vi "HH_Init.vi"(0 "MAXDEV":i32=8, 11 "error in (no error)":errorcluster) -> (4 "Library Version":string="2.1", 6 "Device List":T1(array[cluster]), 15 "error out":errorcluster)   [LabVIEW 2013]
doc: "Prepare PicoHarp 300 for T3R-Measurement"
uses:
  MT Scan/SubVIs/hhlib.dll
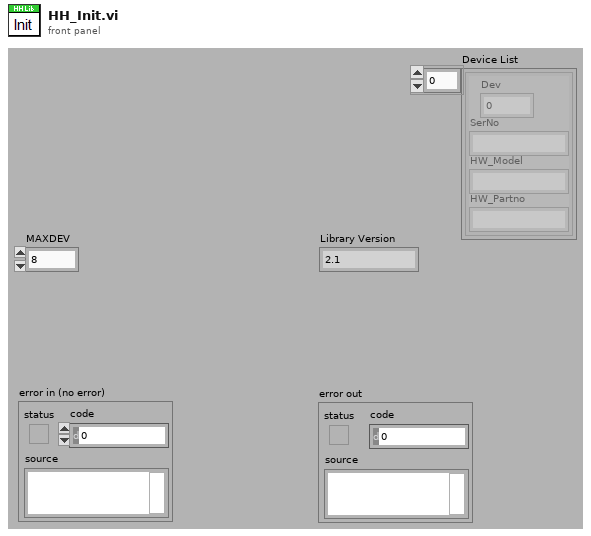
[diagram p1: front panel]
types:
  T1 = cluster{"Dev":i32, "SerNo":string, "HW_Model":string, "HW_Partno":string}[]
  T2 = cluster{"Dev":i32, "SerNo":string, "HW_Model":string, "HW_Partno":string}
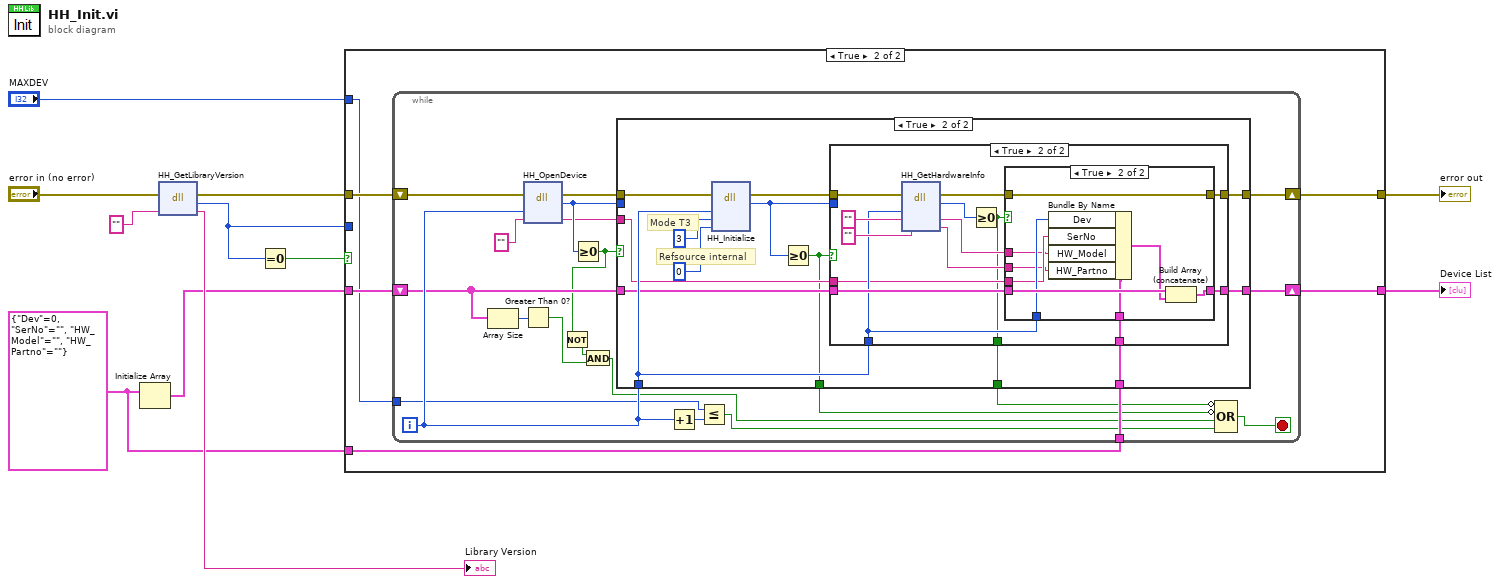
[diagram p0: block diagram]
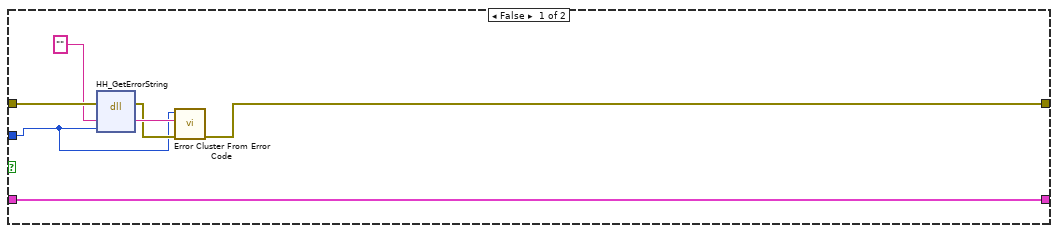
[diagram p2: hidden frame]
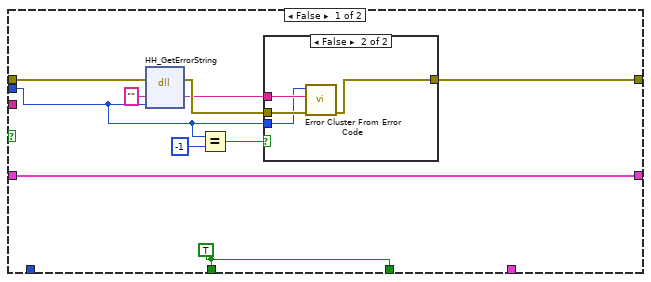
[diagram p3: hidden frame]
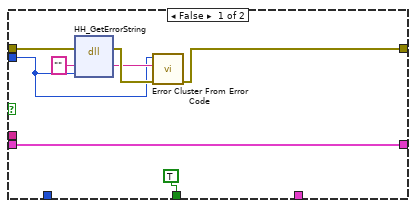
[diagram p5: hidden frame]
diagram:
  w2 = T2 {"Dev"=0, "SerNo"="", "HW_Model"="", "HW_Partno"=""}
  n1 = Initialize Array(w2) -> (w3:T1)  [unwired: 1 in]
  n2 = dll-call lib="C:/Users/dhaehnel/Documents/Workspace/Labview_Workspace/newCore/MT Scan/SubVIs/hhlib.dll" fn="HH_GetLibraryVersion"(error in="error in (no error)", "vers"="") -> (error out=w8:errorcluster, "return type"=w4:i32, "vers"=→"Library Version":string)  [unwired: 2 in, 1 out]
  n3 = Equal To 0?(x=w4) -> (x = 0?=w5:bool)
  n4 = case shown="True" w5 {
    tunnel: w8 -> [w18 w24]
    tunnel: "MAXDEV" -> [_ w19]
    tunnel: [w15 w23] -> w6
    tunnel: w4 -> [w12 _]
    tunnel: w3 -> [w13 w22]
    tunnel: w2 -> [_ w21]
    tunnel: [w13 w20] -> w1
    frame False {
      n5 = dll-call lib="C:/Users/dhaehnel/Documents/Workspace/Labview_Workspace/newCore/MT Scan/SubVIs/hhlib.dll" fn="HH_GetErrorString"(error in=w18, "errstring"="", "errcode"=w12) -> (error out=w16:errorcluster, "errstring"=w17:string)  [unwired: 4 in, 1 out]
      n6 = call <vilib>:"Error Cluster From Error Code.vi"("error in (no error)"=w16, "error message (\"\")"=w17, "error code (0)"=w12) -> ("error out"=w15:errorcluster)  [unwired: 6 in]
    }
    frame True {
      n7 = while {
        shift-right: [w41] -> w23
        shift-left: w24 -> [w45]
        shift-right: [w39] -> w20
        shift-left: w22 -> [w30]
        tunnel: w21 -> [w38]
        tunnel: w19 -> [w34]
        i -> [w36]
        stop <- w37 stop-if-true
        n8 = Array Size(array=w30) -> (size(s)=w29:i32)
        n9 = Greater Than 0?(x=w29) -> (x > 0?=w28:bool)
        n10 = dll-call lib="C:/Users/dhaehnel/Documents/Workspace/Labview_Workspace/newCore/MT Scan/SubVIs/hhlib.dll" fn="HH_OpenDevice"(error in=w45, "devidx"=w36, "serial"="" ("vers")) -> (error out=w43:errorcluster, "return type"=w42:i32, "serial"=w40:string)  [unwired: 3 in, 1 out]
        n11 = Greater Or Equal To 0?(x=w42) -> (x >= 0?=w26:bool)
        n12 = Not(x=w26) -> (.not. x?=w27:bool)
        n13 = And(x=w27, y=w28) -> (x .and. y?=w25:bool)
        n14 = case shown="True" w26 {
          tunnel: w43 -> [w50 w73]
          tunnel: w36 -> [_ w68]
          tunnel: w42 -> [w46 _]
          tunnel: [w55 w69] -> w41
          tunnel: w40 -> [_ w64]
          tunnel: w30 -> [w54 w67]
          tunnel: [w54 w66] -> w39
          tunnel: w38 -> [_ w65]
          tunnel: [w53 w63] -> w32
          tunnel: [w53 w62] -> w31
          frame False {
            w53 = TRUE
            n15 = dll-call lib="C:/Users/dhaehnel/Documents/Workspace/Labview_Workspace/newCore/MT Scan/SubVIs/hhlib.dll" fn="HH_GetErrorString"(error in=w50, "errstring"="", "errcode"=w46) -> (error out=w49:errorcluster, "errstring"=w47:string)  [unwired: 4 in, 1 out]
            n16 = Equal?(x=w46, y=-1) -> (x = y?=w51:bool)
            n17 = case shown="False" w51 {
              tunnel: w47 -> [_ w60]
              tunnel: w49 -> [w56 w59]
              tunnel: [w56 w58] -> w55
              tunnel: w46 -> [_ w57]
              frame True {
              }
              frame False {
                n18 = call <vilib>:"Error Cluster From Error Code.vi"("error in (no error)"=w59, "error message (\"\")"=w60, "error code (0)"=w57) -> ("error out"=w58:errorcluster)  [unwired: 6 in]
              }
            }
          }
          frame True {
            # "Refsource internal"
            # "Mode T3"
            n19 = dll-call lib="C:/Users/dhaehnel/Documents/Workspace/Labview_Workspace/newCore/MT Scan/SubVIs/hhlib.dll" fn="HH_Initialize"(error in=w73, "devidx"=w68, "mode"=3, "refsource"=0) -> (error out=w71:errorcluster, "return type"=w70:i32)  [unwired: 5 in, 1 out]
            n20 = Greater Or Equal To 0?(x=w70) -> (x >= 0?=w63:bool)
            n21 = case shown="True" w63 {
              tunnel: w71 -> [w78 w95]
              tunnel: w70 -> [w74 _]
              tunnel: [w81 w92] -> w69
              tunnel: w68 -> [_ w86]
              tunnel: w67 -> [w80 w89]
              tunnel: [w80 w88] -> w66
              tunnel: w65 -> [_ w87]
              tunnel: w64 -> [_ w85]
              tunnel: [TRUE w82] -> w62
              frame False {
                n22 = dll-call lib="C:/Users/dhaehnel/Documents/Workspace/Labview_Workspace/newCore/MT Scan/SubVIs/hhlib.dll" fn="HH_GetErrorString"(error in=w78, "errstring"="", "errcode"=w74) -> (error out=w77:errorcluster, "errstring"=w76:string)  [unwired: 4 in, 1 out]
                n23 = call <vilib>:"Error Cluster From Error Code.vi"("error in (no error)"=w77, "error message (\"\")"=w76, "error code (0)"=w74) -> ("error out"=w81:errorcluster)  [unwired: 6 in]
              }
              frame True {
                n24 = dll-call lib="C:/Users/dhaehnel/Documents/Workspace/Labview_Workspace/newCore/MT Scan/SubVIs/hhlib.dll" fn="HH_GetHardwareInfo"(error in=w95, "devidx"=w86, "model"="", "partno"="" ("version")) -> (error out=w93:errorcluster, "return type"=w94:i32, "model"=w83:string, "partno"=w84:string)  [unwired: 3 in, 1 out]
                n25 = Greater Or Equal To 0?(x=w94) -> (x >= 0?=w82:bool)
                n26 = case shown="True" w82 {
                  tunnel: w93 -> [w97 w106]
                  tunnel: [w97 w106] -> w92
                  tunnel: w89 -> [w96 w105]
                  tunnel: [w96 w104] -> w88
                  tunnel: w87 -> [_ w103]
                  tunnel: w86 -> [_ w101]
                  tunnel: w85 -> [_ w100]
                  tunnel: w84 -> [_ w99]
                  tunnel: w83 -> [_ w98]
                  frame False {
                  }
                  frame True {
                    n27 = Bundle By Name(cluster=w103, "Dev"=w101, "SerNo"=w100, "HW_Model"=w98, "HW_Partno"=w99) -> (w102:T2)
                    n28 = Build Array (concatenate)(w105, w102) -> (w104:T1)
                  }
                }
              }
            }
          }
        }
        n29 = Increment(x=w36) -> (x+1=w35:i32)
        n30 = Less Or Equal?(x=w34, y=w35) -> (x <= y?=w33:bool)
        n31 = Compound Arithmetic op=OR(invert w31, invert w32, w25, w33) -> (w37:bool)
      }
    }
  }
  "error out" <- w6
  "Device List" <- w1
